vi "Test Air Leak ODBC.vi"() -> ()   [LabVIEW 2013]
uses:
  Controls/ALTS-2015 Obtain Test Data DB Driver Options.ctl
  Controls/ALTS-2015 Station Cluster.ctl
  Controls/ALTS-2015 LV2GBL Options.ctl
panel:
  out "error out":errorcluster
  out "data":string[][](array[string])=[["H                   "], ["1097005             "], ["Sensor 030          "], ["82.887222"], ["79.596405"], ["-0.676844"], ["Pass                                    "], ["9/9/2014 9:59:34 AM "], ["TR001-099289.csv                                  "], ["0"], ["0"], ["41891.4163657407"]]
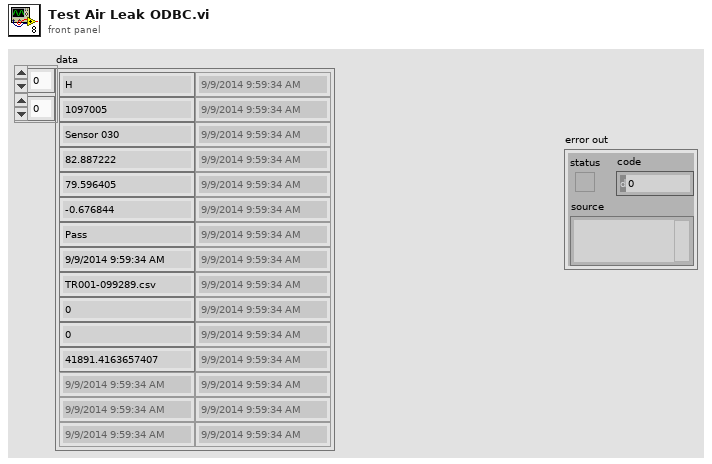
[diagram p1: front panel]
types:
  T1 = typedef "ALTS-2015 LV2GBL Options.ctl" = enum16{"Read all", "Write all"}
  T2 = typedef "ALTS-2015 Station Cluster.ctl" = enum16{"Station 1", "Station 2", "Station 3", "Station 4"}
  T3 = typedef "ALTS-2015 Obtain Test Data DB Driver Options.ctl" = enum16{"Init", "Read Test Data Results", "Close"}
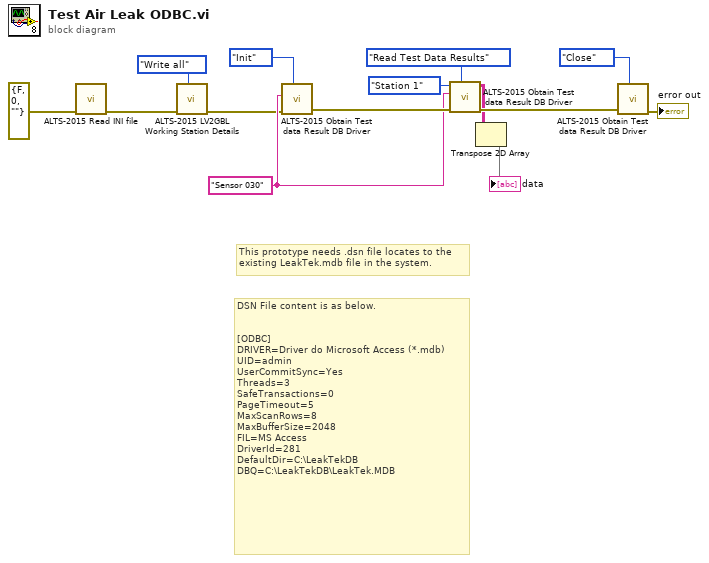
[diagram p0: block diagram]
diagram:
  w8 = "Sensor 030" ("Sensor Name")
  # "DSN File content is as below.\n\n\n[ODBC]\nDRIVER=Driver do Microsoft Access (*.mdb)\nUID=admin\nUserCommitSync=Yes\nThreads=3\nSafeTransactions=0\nPageTimeout=5\nMaxScanRows=8\nMaxBufferSize=2048\nFIL=MS Access\nDriverId=281\nDefaultDir=C:\\LeakTekDB\nDBQ=C:\\LeakTekDB\\LeakTek.MDB"
  # "This prototype needs .dsn file locates to the\nexisting LeakTek.mdb file in the system."
  n1 = call "ALTS-2015 Read INI file.vi"("error in (no error)"=errorcluster {"status"=FALSE, "code"=0, "source"=""} ("error in")) -> ("error out"=w3:errorcluster)  [unwired: 10 in]
  n2 = call "ALTS-2015 LV2GBL Working Station Details.vi"("Options"=ALTS-2015_LV2GBL_Options."Write all", "error in"=w3) -> ("error out"=w2:errorcluster)  [unwired: 8 in, 1 out]
  n3 = call "ALTS-2015 Obtain Test data Result DB Driver.vi"("Option"=ALTS-2015_Obtain_Test_Data_DB_Driver_Options."Init", "error in"=w2, "Sensor Name"=w8) -> ("error out"=w13:errorcluster)  [unwired: 7 in, 1 out]
  n4 = call "ALTS-2015 Obtain Test data Result DB Driver.vi"("Option"=ALTS-2015_Obtain_Test_Data_DB_Driver_Options."Read Test Data Results", "error in"=w13, "Sensor Name"=w8, "Station Enum"=ALTS-2015_Station_Cluster."Station 1") -> ("error out"=w14:errorcluster, "data"=w10:string[][])  [unwired: 6 in]
  n5 = Transpose 2D Array(2D array=w10) -> (transposed array=→"data":string[][])
  n6 = call "ALTS-2015 Obtain Test data Result DB Driver.vi"("Option"=ALTS-2015_Obtain_Test_Data_DB_Driver_Options."Close", "error in"=w14) -> ("error out"=→"error out":errorcluster)  [unwired: 8 in, 1 out]
